vi "流量计全局变量.vi"() -> ()   [LabVIEW 2016, in "流量计.lvlib"]
panel:
  out "通讯包":string
  out "显示值":T1
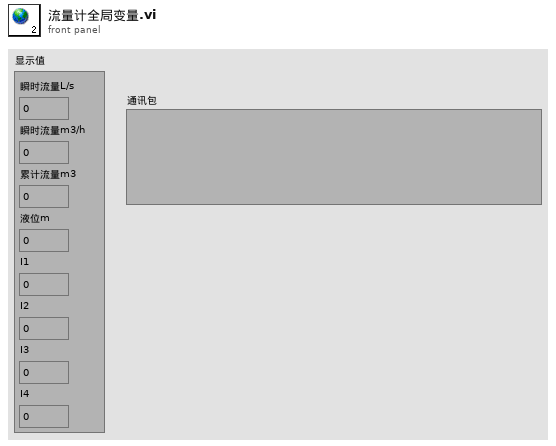
[diagram p1: front panel]
types:
  T1 = cluster{"瞬时流量L/s":dbl, "瞬时流量m3/h":dbl, "累计流量m3":dbl, "液位m":dbl, "I1":dbl, "I2":dbl, "I3":dbl, "I4":dbl}
diagram:
